vi "Generate_Graphs.vi"(4 "Marker 1 Data 2":u8[][][](array[numeric]), 5 "Channel Data":sgl[][][](array[numeric]), 6 "Marker 1 Data":u8[][][](array[numeric]), 7 "Number of Waveforms":i32, 9 "Sample Period (ns)":dbl, 10 "Number to skip":i32=1, 11 "Starting index":i32) -> (0 "Chan4":T3, 1 "Chan3":T3, 2 "Chan2":T3, 3 "Chan1":T3)   [LabVIEW 2010]
panel:
  out "Channel 4,\nAnalog":T1(graph)
  out "Channel 4, \nMarker 1":T2(graph)
  out "Channel 4,\nMarker 2":T2(graph)
  out "Channel 3,\nAnalog":T1(graph)
  out "Channel 3, \nMarker 1":T2(graph)
  out "Channel 1,\nMarker 2":T2(graph)
  out "Channel 2,\nAnalog":T1(graph)
  out "Channel 2, \nMarker 1":T2(graph)
  out "Channel 2,\nMarker 2":T2(graph)
  out "Channel 1,\nAnalog":T1(graph)
  out "Channel 1, \nMarker 1":T2(graph)
  out "Channel 1,\nMarker 2":T2(graph)
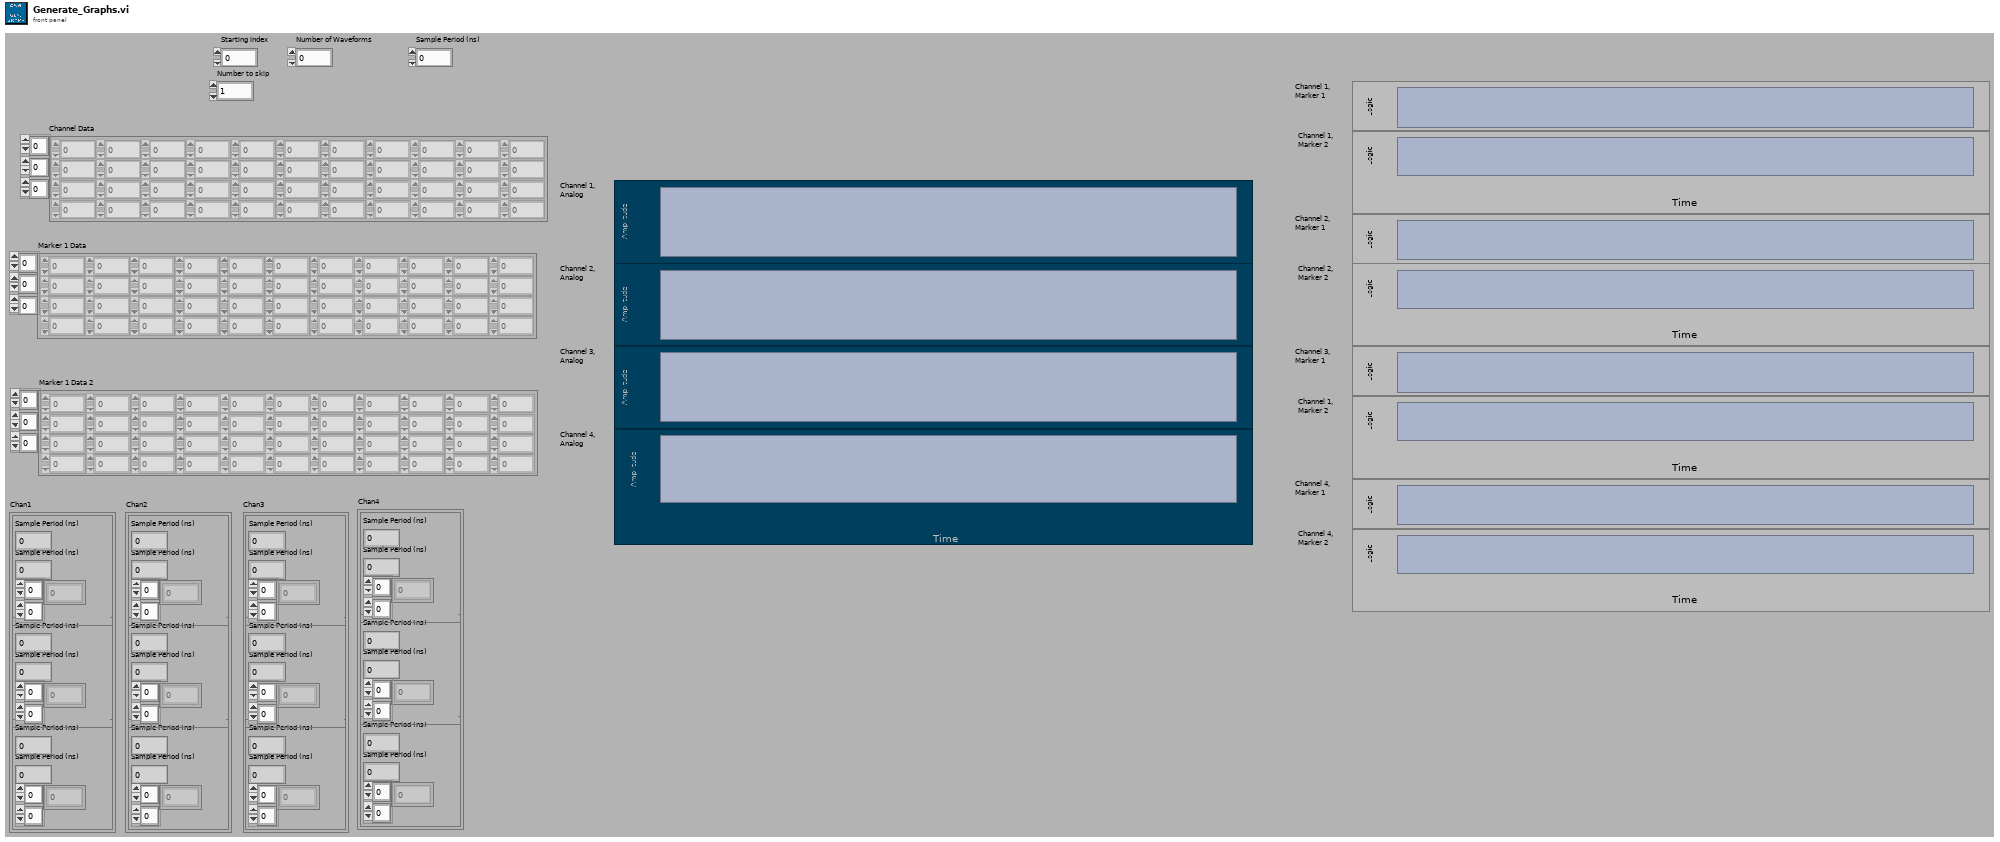
[diagram p1: front panel]
types:
  T1 = cluster{"Sample Period (ns)":dbl, "Sample Period (ns)":dbl, dbl[][]}
  T2 = cluster{"Sample Period (ns)":dbl, "Sample Period (ns)":dbl, u8[][]}
  T3 = cluster{cluster{"Sample Period (ns)":dbl, "Sample Period (ns)":dbl, dbl[][]}, cluster{"Sample Period (ns)":dbl, "Sample Period (ns)":dbl, u8[][]}, cluster{"Sample Period (ns)":dbl, "Sample Period (ns)":dbl, u8[][]}}
  T4 = cluster{dbl[], u8[], u8[], dbl[], u8[], u8[], dbl[], u8[], u8[], dbl[], u8[], u8[]}[]
  T5 = cluster{"Channel Data":sgl[], "Marker 1 Data":u8[], "Marker 1 Data 2":u8[], "Channel Data":sgl[], "Marker 1 Data":u8[], "Marker 1 Data 2":u8[], "Channel Data":sgl[], "Marker 1 Data":u8[], "Marker 1 Data 2":u8[], "Channel Data":sgl[], "Marker 1 Data":u8[], "Marker 1 Data 2":u8[]}
  T6 = cluster{"Channel Data":dbl[], "Marker 1 Data":u8[], "Marker 1 Data 2":u8[], "Channel Data":dbl[], "Marker 1 Data":u8[], "Marker 1 Data 2":u8[], "Channel Data":dbl[], "Marker 1 Data":u8[], "Marker 1 Data 2":u8[], "Channel Data":dbl[], "Marker 1 Data":u8[], "Marker 1 Data 2":u8[]}[]
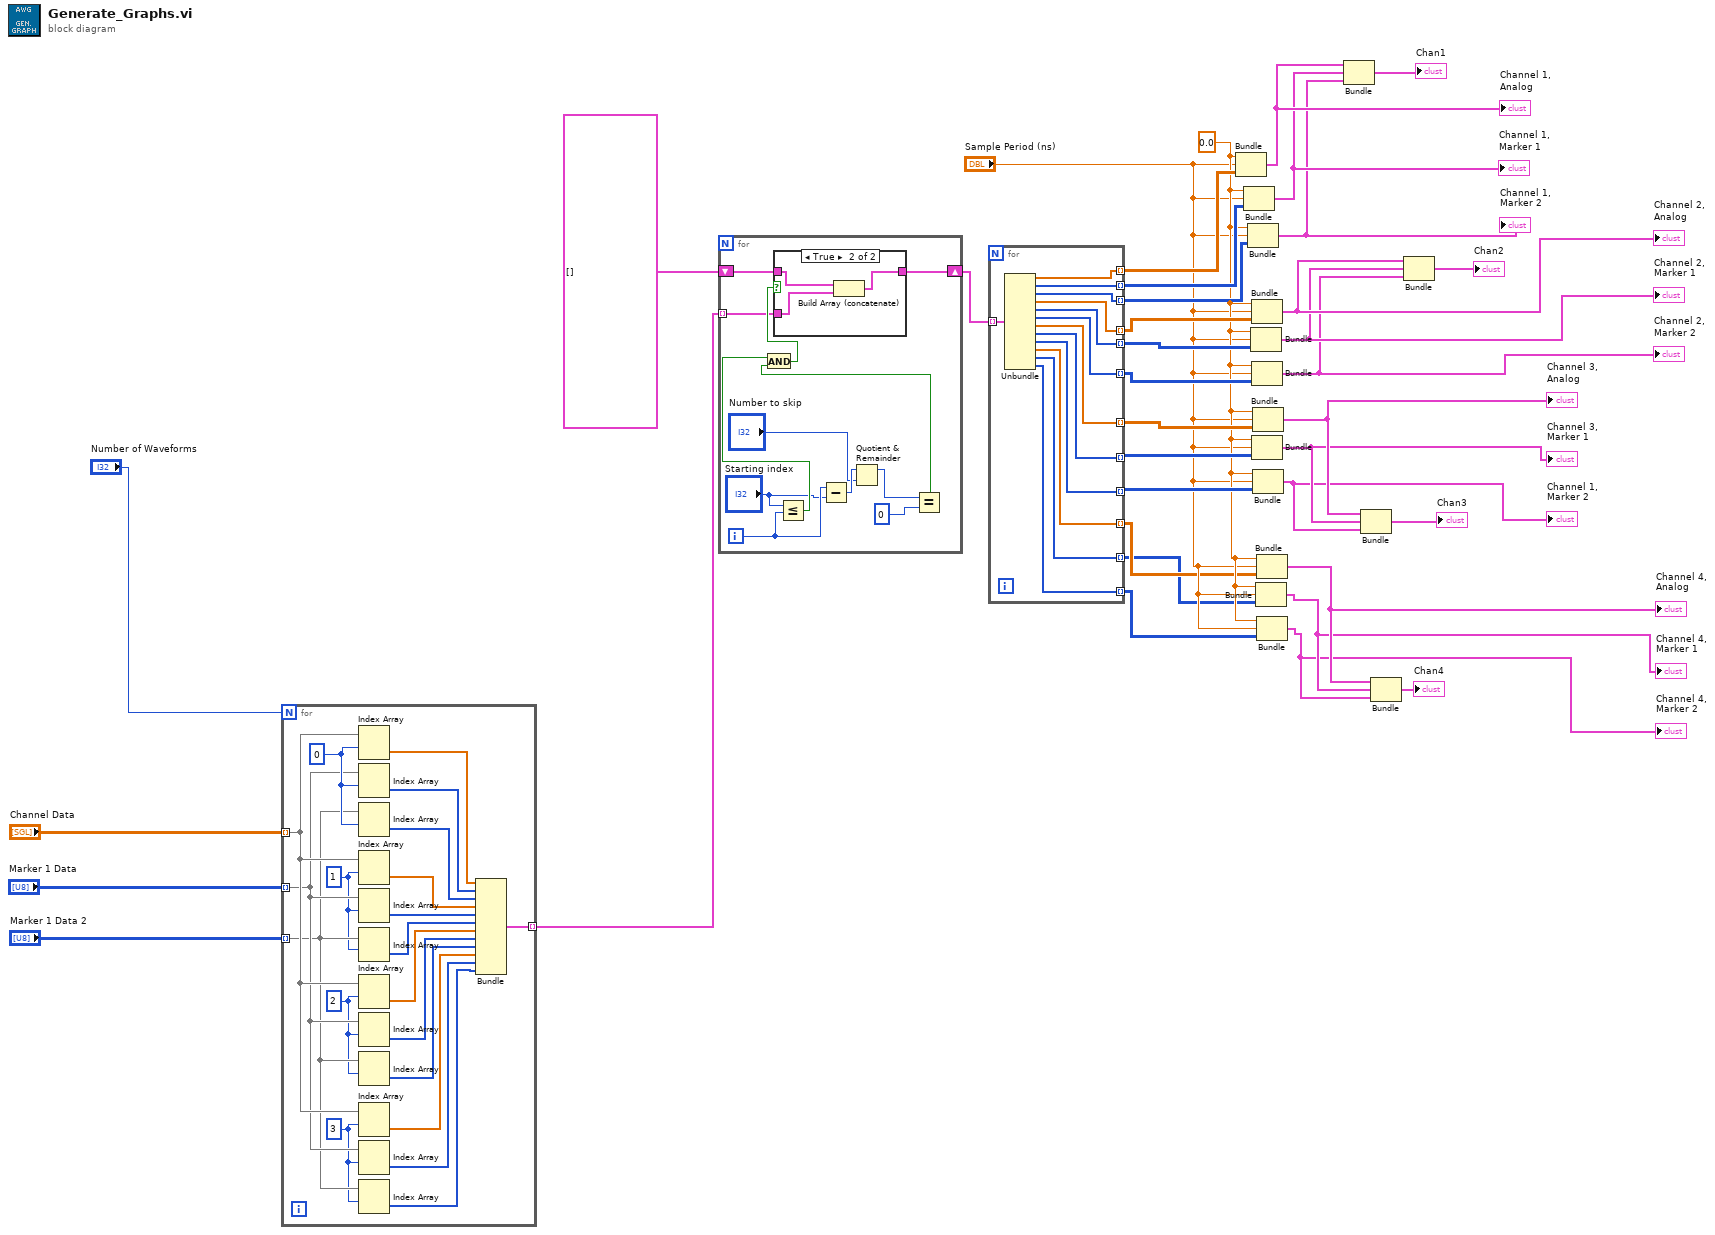
[diagram p0: block diagram]
diagram:
  w23 = 0.0 ("Sample Period (ns)")
  n1 = for {
    N: "Number of Waveforms" -> [_]
    tunnel: "Channel Data" -> [w56] mode=indexing
    tunnel: "Marker 1 Data" -> [w55] mode=indexing
    tunnel: "Marker 1 Data 2" -> [w54] mode=indexing
    tunnel: [w38] -> w11 mode=indexing
    w51 = 3 ("index (row)")
    w52 = 2 ("index (row)")
    w53 = 1 ("index (row)")
    w57 = 0 ("index (row)")
    n2 = Index Array(array=w56, index (row)=w57) -> (element=w50:sgl[])  [unwired: 1 in]
    n3 = Index Array(array=w55, index (row)=w57) -> (element=w49:u8[])  [unwired: 1 in]
    n4 = Index Array(array=w54, index (row)=w57) -> (element=w48:u8[])  [unwired: 1 in]
    n5 = Index Array(array=w56, index (row)=w53) -> (element=w47:sgl[])  [unwired: 1 in]
    n6 = Index Array(array=w55, index (row)=w53) -> (element=w46:u8[])  [unwired: 1 in]
    n7 = Index Array(array=w54, index (row)=w53) -> (element=w45:u8[])  [unwired: 1 in]
    n8 = Index Array(array=w56, index (row)=w52) -> (element=w44:sgl[])  [unwired: 1 in]
    n9 = Index Array(array=w55, index (row)=w52) -> (element=w43:u8[])  [unwired: 1 in]
    n10 = Index Array(array=w54, index (row)=w52) -> (element=w42:u8[])  [unwired: 1 in]
    n11 = Index Array(array=w56, index (row)=w51) -> (element=w41:sgl[])  [unwired: 1 in]
    n12 = Index Array(array=w55, index (row)=w51) -> (element=w40:u8[])  [unwired: 1 in]
    n13 = Index Array(array=w54, index (row)=w51) -> (element=w39:u8[])  [unwired: 1 in]
    n14 = Bundle("Channel Data"=w50, "Marker 1 Data"=w49, "Marker 1 Data 2"=w48, "Channel Data"=w47, "Marker 1 Data"=w46, "Marker 1 Data 2"=w45, "Channel Data"=w44, "Marker 1 Data"=w43, "Marker 1 Data 2"=w42, "Channel Data"=w41, "Marker 1 Data"=w40, "Marker 1 Data 2"=w39) -> (w38:T5)  [unwired: 1 in]
  }
  n15 = for {
    shift-right: [w68] -> w37
    shift-left: T4 [] -> [w69]
    tunnel: w11 -> [w58] mode=indexing
    i -> [w61]
    n16 = Less Or Equal?(x="Starting index", y=w61) -> (x <= y?=w66:bool)
    n17 = Subtract(x=w61, y="Starting index") -> (x-y=w65:i32)
    n18 = Quotient & Remainder(x=w65, y="Number to skip") -> (x-y*floor(x/y)=w59:i32)  [unwired: 1 out]
    n19 = Equal?(x=w59, y=0) -> (x = y?=w62:bool)
    n20 = And(x=w66, y=w62) -> (x .and. y?=w67:bool)
    n21 = case shown="True" w67 {
      tunnel: w69 -> [w70 w73]
      tunnel: [w70 w72] -> w68
      tunnel: w58 -> [_ w71]
      frame False {
      }
      frame True {
        n22 = Build Array (concatenate)(w73, w71) -> (w72:T6)
      }
    }
  }
  n23 = for {
    tunnel: w37 -> [w86] mode=indexing
    tunnel: [w85] -> w35 mode=indexing
    tunnel: [w84] -> w34 mode=indexing
    tunnel: [w83] -> w33 mode=indexing
    tunnel: [w82] -> w29 mode=indexing
    tunnel: [w81] -> w28 mode=indexing
    tunnel: [w80] -> w27 mode=indexing
    tunnel: [w79] -> w26 mode=indexing
    tunnel: [w78] -> w25 mode=indexing
    tunnel: [w77] -> w24 mode=indexing
    tunnel: [w76] -> w21 mode=indexing
    tunnel: [w75] -> w19 mode=indexing
    tunnel: [w74] -> w20 mode=indexing
    n24 = Unbundle(w86) -> (w85:dbl[], w84:u8[], w83:u8[], w82:dbl[], w81:u8[], w80:u8[], w79:dbl[], w78:u8[], w77:u8[], w76:dbl[], w75:u8[], w74:u8[])
  }
  n25 = Bundle("Sample Period (ns)"=w23, "Sample Period (ns)"="Sample Period (ns)", w35) -> (w32:T1)  [unwired: 1 in]
  "Channel 1,\nAnalog" <- w32
  n26 = Bundle("Sample Period (ns)"=w23, "Sample Period (ns)"="Sample Period (ns)", w34) -> (w31:T2)  [unwired: 1 in]
  "Channel 1, \nMarker 1" <- w31
  n27 = Bundle("Sample Period (ns)"=w23, "Sample Period (ns)"="Sample Period (ns)", w33) -> (w30:T2)  [unwired: 1 in]
  "Channel 1,\nMarker 2" <- w30
  n28 = Bundle("Sample Period (ns)"=w23, "Sample Period (ns)"="Sample Period (ns)", w28) -> (w6:T2)  [unwired: 1 in]
  "Channel 2, \nMarker 1" <- w6
  n29 = Bundle("Sample Period (ns)"=w23, "Sample Period (ns)"="Sample Period (ns)", w29) -> (w7:T1)  [unwired: 1 in]
  "Channel 2,\nAnalog" <- w7
  n30 = Bundle("Sample Period (ns)"=w23, "Sample Period (ns)"="Sample Period (ns)", w27) -> (w5:T2)  [unwired: 1 in]
  "Channel 2,\nMarker 2" <- w5
  n31 = Bundle("Sample Period (ns)"=w23, "Sample Period (ns)"="Sample Period (ns)", w25) -> (w9:T2)  [unwired: 1 in]
  "Channel 3, \nMarker 1" <- w9
  n32 = Bundle("Sample Period (ns)"=w23, "Sample Period (ns)"="Sample Period (ns)", w26) -> (w10:T1)  [unwired: 1 in]
  "Channel 3,\nAnalog" <- w10
  n33 = Bundle("Sample Period (ns)"=w23, "Sample Period (ns)"="Sample Period (ns)", w24) -> (w8:T2)  [unwired: 1 in]
  "Channel 1,\nMarker 2" <- w8
  n34 = Bundle("Sample Period (ns)"=w23, "Sample Period (ns)"="Sample Period (ns)", w19) -> (w3:T2)  [unwired: 1 in]
  "Channel 4, \nMarker 1" <- w3
  n35 = Bundle("Sample Period (ns)"=w23, "Sample Period (ns)"="Sample Period (ns)", w21) -> (w4:T1)  [unwired: 1 in]
  "Channel 4,\nAnalog" <- w4
  n36 = Bundle("Sample Period (ns)"=w23, "Sample Period (ns)"="Sample Period (ns)", w20) -> (w2:T2)  [unwired: 1 in]
  "Channel 4,\nMarker 2" <- w2
  n37 = Bundle(w32, w31, w30) -> (→"Chan1":T3)  [unwired: 1 in]
  n38 = Bundle(w10, w9, w8) -> (→"Chan3":T3)  [unwired: 1 in]
  n39 = Bundle(w4, w3, w2) -> (→"Chan4":T3)  [unwired: 1 in]
  n40 = Bundle(w7, w6, w5) -> (→"Chan2":T3)  [unwired: 1 in]
